vi "SendAndAskForReply.vi"(6 "Delay between send and receive [ms]":i32, 7 "timeout for sending data [ms]":i32=5000, 8 "error in (no error)":errorcluster, 9 "timeout for receiving data [ms]":i32=5000, 10 "String to be sent":string="{\"id\":1234, \"command\":\"icl_info\"}", 11 "Communicator in":refnum<class "Communicator.lvclass">) -> (0 "error out":errorcluster, 2 "Data":string, 3 "Communicator out":refnum<class "Communicator.lvclass">)   [LabVIEW 2023, in "Communicator.lvclass"]
doc: "Wrapper around send and receive for the websocket communication."
uses:
  Communicator.lvclass
  Communicator.lvclass/Communicator.ctl
  fd4945cd-9c85-4faf-8cc2-4a6213abe34b.vi
  <vilib>/Hampel Software Engineering/HSE Logger/hse-logger.lvlib
  <vilib>/JDP Science/JSONtext/JSONtext.lvlib
panel:
  # "Connector Pane"
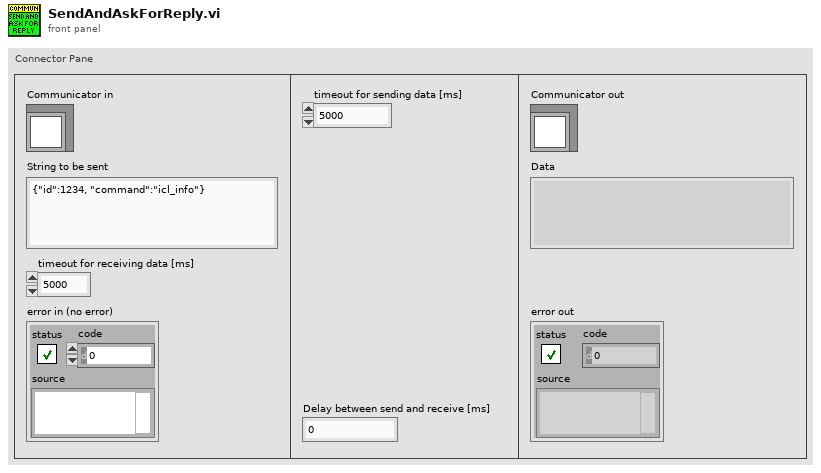
[diagram p1: front panel]
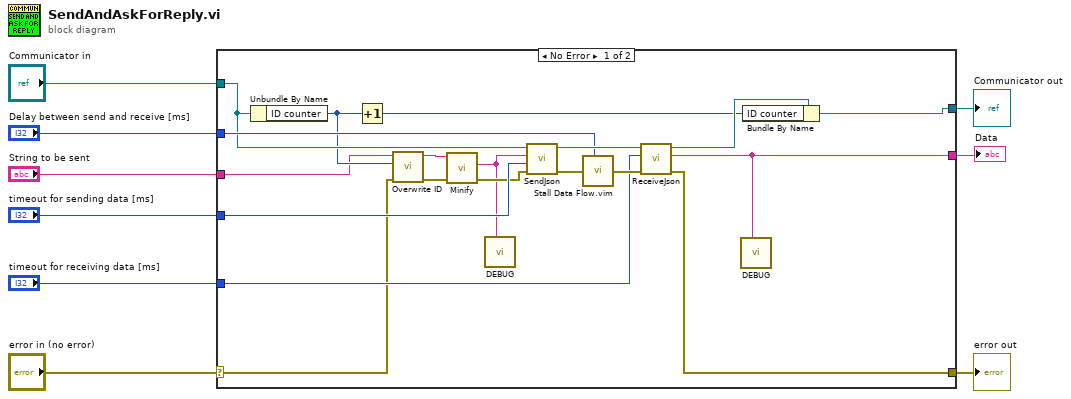
[diagram p0: block diagram]
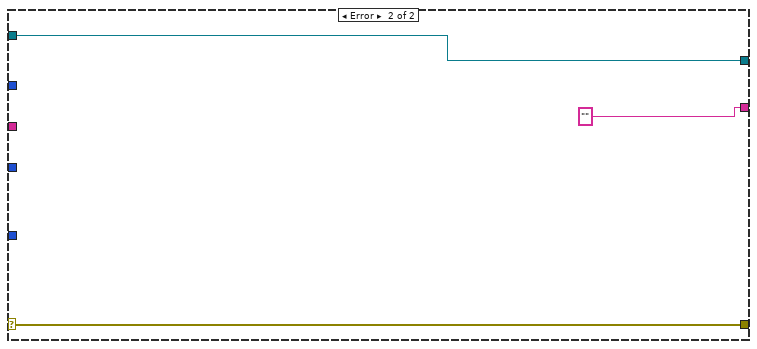
[diagram p2: hidden frame]
diagram:
  n1 = case shown="No Error" "error in (no error)" {
    selector: "error in (no error)" -> [w15 w30]
    tunnel: [w25 w30] -> w9
    tunnel: [w16 w29] -> w7
    tunnel: "Communicator in" -> [w20 w29]
    tunnel: "Delay between send and receive [ms]" -> [w21 _]
    tunnel: "timeout for sending data [ms]" -> [w24 _]
    tunnel: "String to be sent" -> [w10 _]
    tunnel: [w13 "" ("Data")] -> w4
    tunnel: "timeout for receiving data [ms]" -> [w23 _]
    frame No Error {
      n2 = Unbundle By Name(w20) -> ("ID counter"=w18:i32)
      n3 = Increment(x=w18) -> (x+1=w17:i32)
      n4 = call "Overwrite ID.vi"("error in (no error)"=w15, "Numeric"=w18, "String"=w10) -> ("error out"=w14:errorcluster, "<JSON>"=w12:string)  [unwired: 7 in]
      n5 = call <vilib>:"Minify.vi"("JSON"=w12) -> ("Rest of Input String"=w11:string)  [unwired: 8 in, 2 out]
      n6 = call <vilib>:"DEBUG.vi"("Message"=w11) -> ()  [unwired: 10 in, 1 out]
      n7 = call-dynamic "SendJson.vi"("error in (no error)"=w14, "timeout"=w24, "String Data"=w11, "Communicator in"=w20) -> ("error out"=w26:errorcluster, "Communicator out"=w22:refnum<class "Communicator.lvclass">)  [unwired: 6 in]
      n8 = call "Stall Data Flow.vim"("value in"=w26, "milliseconds to wait"=w21) -> ("value out"=w27:errorcluster)  [unwired: 1 out]
      n9 = call-dynamic "ReceiveJson.vi"("error in (no error)"=w27, "timeout [ms]"=w23, "Communicator in"=w22) -> ("error out"=w25:errorcluster, "Data"=w13:string, "Communicator out"=w19:refnum<class "Communicator.lvclass">)  [unwired: 6 in]
      n10 = call <vilib>:"DEBUG.vi"("Message"=w13) -> ()  [unwired: 10 in, 1 out]
      n11 = Bundle By Name(cluster=w19, "ID counter"=w17) -> (w16:refnum<class "Communicator.lvclass">)
    }
    frame Error {
    }
  }
  "error out" <- w9
  "Communicator out" <- w7
  "Data" <- w4
